vi "Do.vi"(8 "error in":errorcluster, 10 "Actor in":refnum<class "Actor.lvclass">, 11 "Get Serialized Device Configuration MSG":refnum<class "Get Serialized Device Configuration MSG.lvclass">) -> (0 "error out":errorcluster, 2 "Actor out":refnum<class "Actor.lvclass">)   [LabVIEW 2014, in "Controller.lvlib" / "Get Serialized Device Configuration MSG.lvclass"]
doc: "(<B>Filename</B>: Actor Framework.lvlib:Message.lvclass:Do.vi)\n\nDefines what a message does when it is received by an actor. Generally, a message instructs an actor to invoke one of its methods. By default, this method does nothing. A child class must override it to define behavior. Create a child class by using the Actor Framework Message Maker dialog box."
uses:
  Get Serialized Device Configuration MSG.lvclass
  <vilib>/ActorFramework/Actor/Actor.lvclass
  Get Serialized Device Configuration MSG.lvclass/Get Serialized Device Configuration MSG.ctl
  reusable/DAQ Device/DAQ Device.lvlib
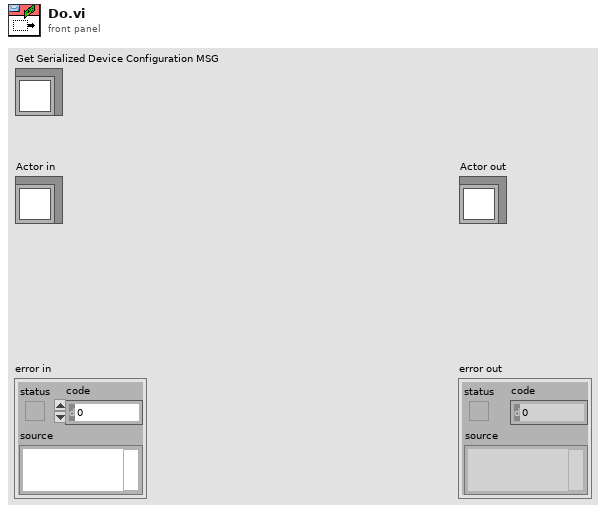
[diagram p1: front panel]
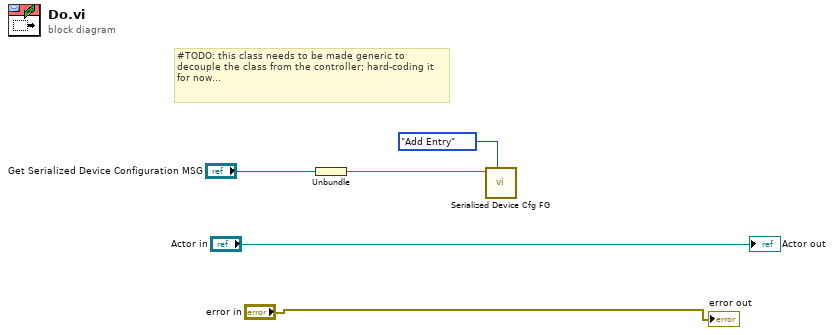
[diagram p0: block diagram]
diagram:
  # "#TODO: this class needs to be made generic to decouple the class from the controller; hard-coding it for now..."
  n1 = Unbundle("Get Serialized Device Configuration MSG") -> (w2:string)
  n2 = call "Serialized Device Cfg FG.vi"("State"=enum16{"Add Entry", "Init", "Get"}."Add Entry", "CfgStrIn"=w2) -> ()  [unwired: 9 in, 1 out]
  "error out" <- "error in"
  "Actor out" <- "Actor in"
